vi "LimitVerticalRange.vi"(8 "error in":errorcluster, 9 "Bottom of Range":i32=480, 10 "Top of Range":i32, 11 "Image":T1) -> (0 "error out":errorcluster, 3 "Image Out":T1)   [LabVIEW 2013]
uses:
  <vilib>/vision/Image Controls.llb/IMAQ Image.ctl
  <vilib>/vision/NI_Vision_Development_Module.lvlib
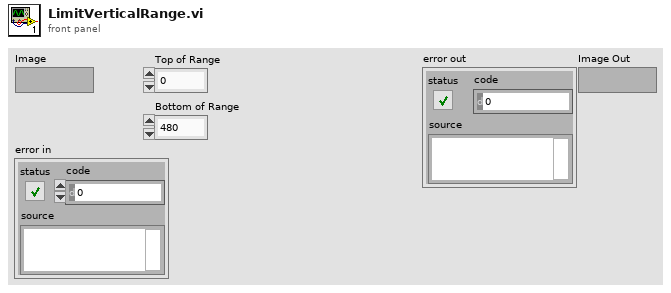
[diagram p1: front panel]
types:
  T1 = typedef "IMAQ Image.ctl" = refnum<image>
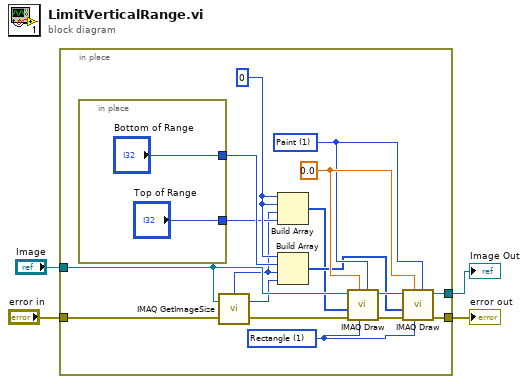
[diagram p0: block diagram]
diagram:
  n1 = in-place {
    in-place-border: [w20] -> w1
    in-place-border: [w15] -> w2
    in-place-border: "error in" -> [w14]
    in-place-border: "Image" -> [w12]
    w10 = 0
    w17 = u16 1 items=["Line", "Rectangle", "Oval"] ("Shape to draw")
    w19 = sgl 0.0 ("Pixel Color")
    w18 = u16 1 items=["Frame", "Paint", "Invert Frame", "Invert Paint"] ("Draw Mode")
    n2 = in-place {
      in-place-border: ["Bottom of Range"] -> w11
      in-place-border: ["Top of Range"] -> w9
    }
    n3 = call "IMAQ GetImageSize"("Image"=w12, "error in (no error)"=w14) -> ("Y Resolution"=w7:i32, "X Resolution"=w8:i32, "error out"=w13:errorcluster)  [unwired: 2 in]
    n4 = Build Array(w10, w10, w8, w9) -> (w5:i32[])
    n5 = Build Array(w10, w11, w8, w7) -> (w6:i32[])
    n6 = call "IMAQ Draw"("Draw Mode"=w18, "Shape to draw"=w17, "Pixel Color"=w19, "error in (no error)"=w13, "Coordinates"=w5, "Image Src"=w12) -> ("error out"=w16:errorcluster, "Image Dst Out"=w21:T1)  [unwired: 4 in]
    n7 = call "IMAQ Draw"("Draw Mode"=w18, "Shape to draw"=w17, "Pixel Color"=w19, "error in (no error)"=w16, "Coordinates"=w6, "Image Src"=w21) -> ("error out"=w15:errorcluster, "Image Dst Out"=w20:T1)  [unwired: 4 in]
  }
  "error out" <- w2
  "Image Out" <- w1
